vi "Create Plugin Groups.vi"(8 "error in (no error)":errorcluster, 9 "String":string, 10 "dsf refnum in":T1, 11 "Section Ptr":T2 format="%.0x") -> (0 "error out":errorcluster)   [LabVIEW 2017, in "Data Sharing Framework System Explorer.lvlib"]
uses:
  Data Sharing Framework System Explorer.lvlib
  <vilib>/NI Veristand/Custom Device API/Custom Device Item Ref.ctl
  dsf core/Source/DSF Configuration API/1.0.0/Public/Controls/DSF Config Data RefNum.ctl
  dsf core/Source/DSF Configuration API/1.0.0/Public/Read Item Child IDs/Read Plugin Group IDs.vi
  dsf core/Source/DSF Configuration API/1.0.0/Public/Read Item/Read Group.vi
  <vilib>/NI VeriStand/Custom Device API/Custom Device API.lvlib
  dsf core/Source/DSF Configuration API/1.0.0/DSF Configuration API.lvlib
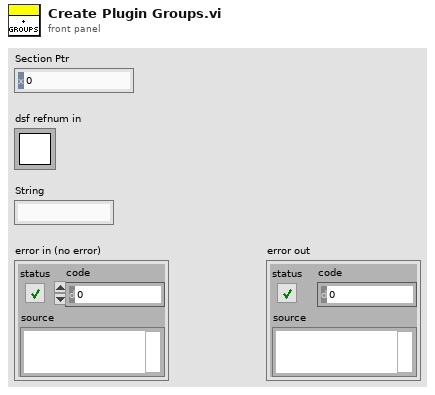
[diagram p1: front panel]
types:
  T1 = typedef "DSF Configuration API.lvlib/DSF Config Data RefNum.ctl" = refnum<k1>
  T2 = typedef "Custom Device API.lvlib/Custom Device Item Ref.ctl" = u64
  T3 = typedef "DSF Configuration API.lvlib/DSF Group Info.ctl" = cluster{"direction":T4, "timing":T5, "transfer ids":string[], "settings id":string}
  T4 = typedef "DSF Configuration API.lvlib/DSF Direction.ctl" = enum8{"Tx", "Rx"}
  T5 = typedef "DSF Configuration API.lvlib/DSF Timing Info.ctl" = cluster{"priority":u64, "decimation":u64, "offset":u64}
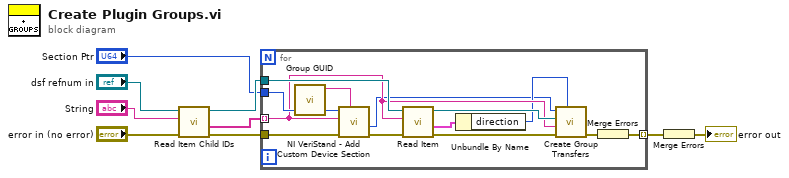
[diagram p0: block diagram]
diagram:
  n1 = call-poly "Read Item Child IDs.vi"("error in (no error)"="error in (no error)", "Plugin ID"="String", "dsf refnum"="dsf refnum in") -> ("error out"=w2:errorcluster, "Group IDs"=w1:string[], "dsf refnum out"=w8:T1)  [unwired: 5 in, 1 out]
  n2 = for {
    tunnel: w1 -> [w14] mode=indexing
    tunnel: "Section Ptr" -> [w22]
    tunnel: w2 -> [w21]
    tunnel: [w19] -> w6 mode=indexing
    tunnel: w8 -> [w17]
    n3 = call "Group GUID.vi"() -> ("GUID"=w10:string)  [unwired: 11 in]
    n4 = call <vilib>:"NI VeriStand - Add Custom Device Section.vi"("GUID (Default Section)"=w10, "error in (no error)"=w21, "Section Name"=w14, "Parent Ref in"=w22) -> ("error out"=w20:errorcluster, "Section Ptr"=w11:T2)  [unwired: 4 in, 2 out]
    n5 = call-poly "Read Item.vi"("error in (no error)"=w20, "Group ID"=w14, "dsf refnum"=w17) -> ("error out"=w18:errorcluster, "value"=w15:T3, "dsf refnum out"=w16:T1)  [unwired: 5 in, 1 out]
    n6 = Unbundle By Name(w15) -> ("direction"=w13:T4)
    n7 = call "Create Group Transfers.vi"("direction"=w13, "error in (no error)"=w18, "Group ID"=w14, "dsf refnum in"=w16, "Section Ptr"=w11) -> ("error out"=w12:errorcluster)  [unwired: 6 in]
    n8 = Merge Errors(w12) -> (w19:errorcluster)
  }
  n9 = Merge Errors(w6) -> (→"error out":errorcluster)
